vi "Pixel_LIDAR_Run.vi"(1 "Noise (0.1 to 1)":dbl, 4 "Initial\nSonarRay\nArray":i32[](array[numeric]), 5 "error in (no error)":errorcluster, 6 "SonarRange":dbl=20.0 min=20.0 max=300.0, 7 "NumberOfBeams":i32=1 min=1 max=360 step=1, 8 "SubPosition":T2, 9 "MDF Image In":T1) -> (0 "error out":errorcluster, 2 "Collision\nWarning":bool, 3 "Sonar Data (r:pixel b:degrees)":cluster{"Range":dbl, "Bearing":dbl}[](array[cluster]))   [LabVIEW 2012]
doc: "This SubVI takes the TunaSub's current position and heading and MDF and calculates the sonar range to shore along a set of evenly spaced sonar rays over a fixed sensor range.\nIt looks for the pixel color change from blue (255) to anything to calculate range."
uses:
  <vilib>/vision/Image Controls.llb/IMAQ Image.ctl
  <vilib>/vision/NI_Vision_Development_Module.lvlib
panel:
  # "This SubVI takes TunaSub's current position and orientaton and MDF and calculates the sonar range to shore along a set of evenly spaced sonar beams (NumberOfBeams) over a fixed sensor range (SonarRange)"
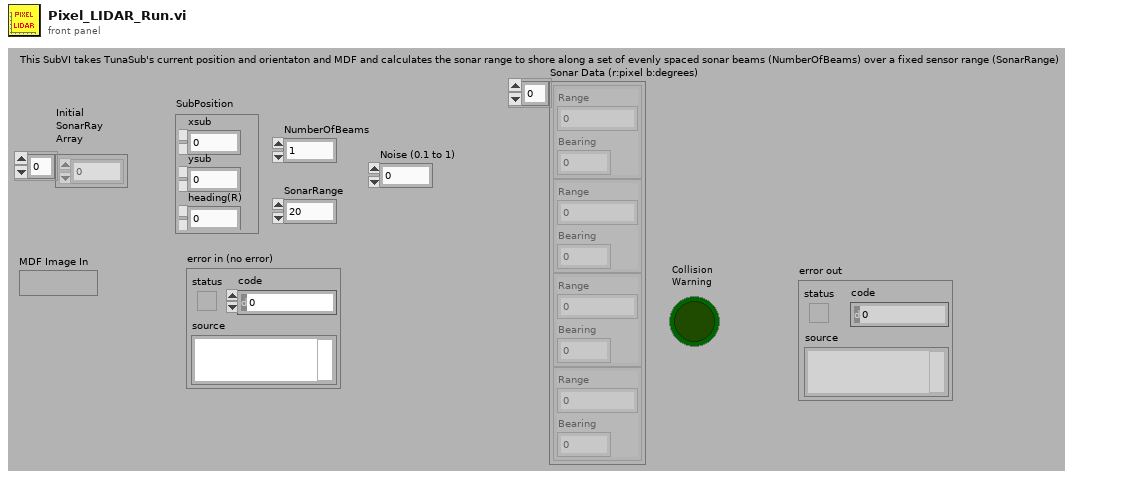
[diagram p1: front panel]
types:
  T1 = typedef "IMAQ Image.ctl" = refnum<image>
  T2 = cluster{"xsub":dbl, "ysub":dbl, "heading(R)":dbl}
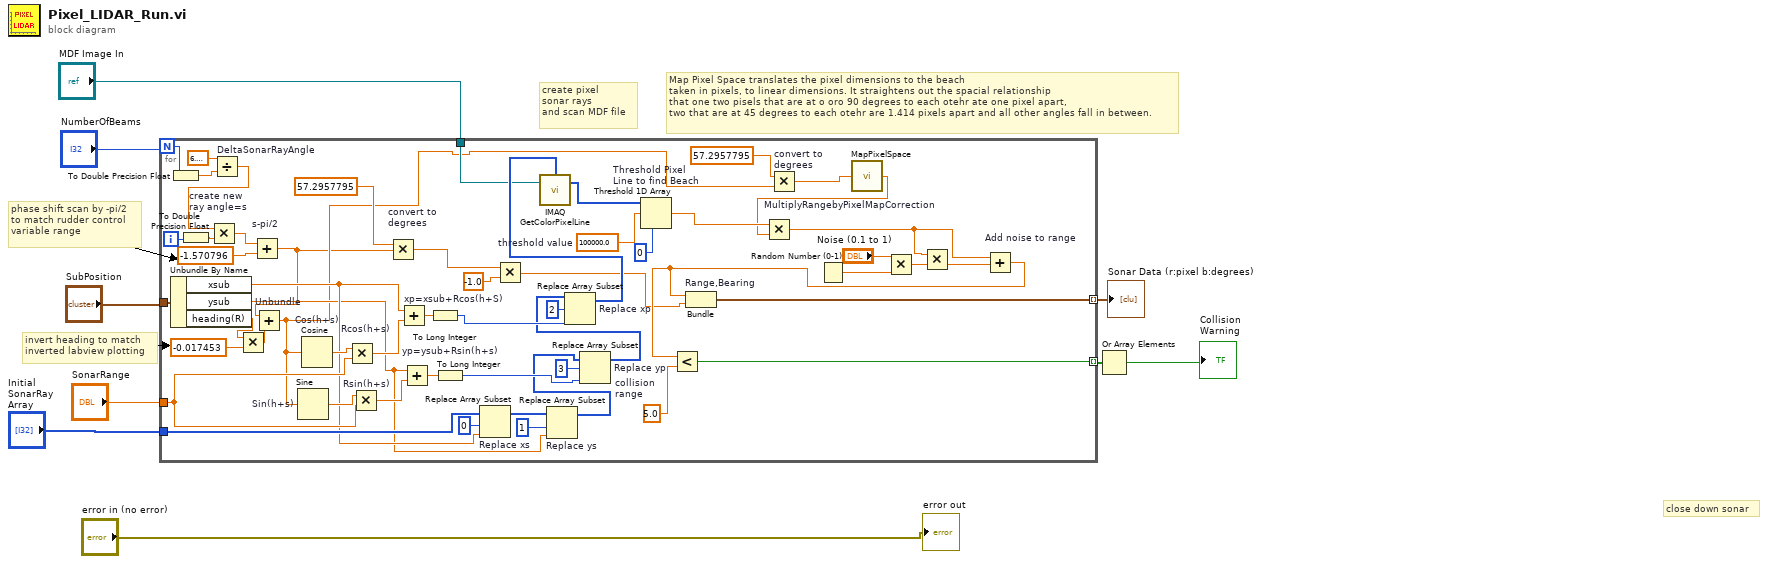
[diagram p0: block diagram]
diagram:
  # "phase shift scan by -pi/2\nto match rudder control\nvariable range"
  # "invert heading to match\ninverted labview plotting"
  # "Map Pixel Space translates the pixel dimensions to the beach\ntaken in pixels, to linear dimensions. It straightens out the spacial relationship \nthat one two pisels that are at o oro 90 degrees to each otehr ate one pixel apart,\ntwo that are at 45 degrees to each otehr are 1.414 pixels apart and all other angles fall in between."
  # "create pixel \nsonar rays\nand scan MDF file"
  # "close down sonar"
  n1 = for {
    N: "NumberOfBeams" -> [w43]
    tunnel: "SonarRange" -> [w61]
    tunnel: "SubPosition" -> [w64]
    tunnel: "MDF Image In" -> [w37]
    tunnel: "Initial\nSonarRay\nArray" -> [w51]
    tunnel: [w34] -> w3 mode=indexing
    tunnel: [w31] -> w2 mode=indexing
    i -> [w39]
    w32 = 5.0  # collision range
    w36 = 100000.0  # threshold value
    n2 = To Double Precision Float(number=w43) -> (double precision float=w41:dbl)
    n3 = Unbundle By Name "Unbundle"(w64) -> ("xsub"=w46:dbl, "ysub"=w45:dbl, "heading(R)"=w17:dbl)
    n4 = To Double Precision Float(number=w39) -> (double precision float=w40:dbl)
    n5 = Divide "DeltaSonarRayAngle"(x=6.283185307179586, y=w41) -> (x/y=w42:dbl)
    n6 = Multiply "create new \nray angle=s"(x=w42, y=w40) -> (x*y=w14:dbl)
    n7 = Multiply(x=w17, y=-0.017453) -> (x*y=w16:dbl)
    n8 = Add "s-pi/2"(x=w14, y=-1.570796) -> (x+y=w13:dbl)
    n9 = Add(x=w13, y=w16) -> (x+y=w26:dbl)
    n10 = Sine "Sin(h+s)"(x=w26) -> (sin(x)=w59:dbl)
    n11 = Cosine "Cos(h+s)"(x=w26) -> (cos(x)=w60:dbl)
    n12 = Multiply "Rcos(h+s)"(x=w60, y=w61) -> (x*y=w63:dbl)
    n13 = Multiply "Rsin(h+s)"(x=w59, y=w61) -> (x*y=w62:dbl)
    n14 = Multiply "convert to\ndegrees"(x=57.2957795 ("y"), y=w13) -> (x*y=w28:dbl)
    n15 = Add "xp=xsub+Rcos(h+S)"(x=w46, y=w63) -> (x+y=w55:dbl)
    n16 = Add "yp=ysub+Rsin(h+s)"(x=w45, y=w62) -> (x+y=w56:dbl)
    n17 = To Long Integer(number=w55) -> (32bit integer=w54:i32)
    n18 = To Long Integer(number=w56) -> (32bit integer=w53:i32)
    n19 = Replace Array Subset "Replace xs"(array=w51, new element=w46, index=0) -> (w50:i32[])
    n20 = Multiply(x=w28, y=-1.0) -> (x*y=w19:dbl)
    n21 = Replace Array Subset "Replace ys"(array=w50, new element=w45, index=1) -> (w49:i32[])
    n22 = Replace Array Subset "Replace yp"(array=w49, new element=w53, index=3) -> (w52:i32[])
    n23 = Replace Array Subset "Replace xp"(array=w52, new element=w54, index=2) -> (w38:i32[])
    n24 = call "IMAQ GetColorPixelLine"("Line Coordinates"=w38, "Image"=w37) -> ("Pixels Line (U32)"=w33:u32[])  [unwired: 2 in, 2 out]
    n25 = Threshold 1D Array "Threshold Pixel\nLine to find Beach"(1:0 ("start index (0)"), 2:w36, 3:w33) -> (0:w29:dbl)
    n26 = Multiply "convert to\ndegrees"(x=57.2957795 ("y"), y=w26) -> (x*y=w11:dbl)
    n27 = Random Number (0-1)() -> (number: 0 to 1=w25:dbl)
    n28 = call "MapPixelSpace.vi"("angle (deg)"=w11) -> ("spacemapout"=w10:dbl)
    n29 = Multiply "MultiplyRangebyPixelMapCorrection"(x=w29, y=w10) -> (x*y=w20:dbl)
    n30 = Multiply ("add noise in")(x="Noise (0.1 to 1)", y=w25) -> (x*y=w23:dbl)
    n31 = Multiply(x=w20, y=w23) -> (x*y=w21:dbl)
    n32 = Add "Add noise to range"(x=w20, y=w21) -> (x+y=w22:dbl)
    n33 = Less?(x=w22, y=w32) -> (x < y?=w31:bool)
    n34 = Bundle "Range,Bearing"(w22, w19) -> (w34:cluster{dbl, dbl})  [unwired: 1 in]
  }
  "Sonar Data (r:pixel b:degrees)" <- w3
  n35 = Or Array Elements(Boolean array=w2) -> (logical OR=→"Collision\nWarning":bool)
  "error out" <- "error in (no error)"
